vi "niRFUtil RFHS Math Complex Magnitude Squared.vi"(0 "data in":csg[](array[numeric]), 2 "RFHS?":bool=TRUE, 7 "result in":sgl[](array[numeric]), 11 "error in":errorcluster) -> (4 "result out":sgl[](array[numeric]), 15 "error out":errorcluster)   [LabVIEW 2015, in "niRFUtil.lvlib"]
uses:
  niRFUtil.lvlib
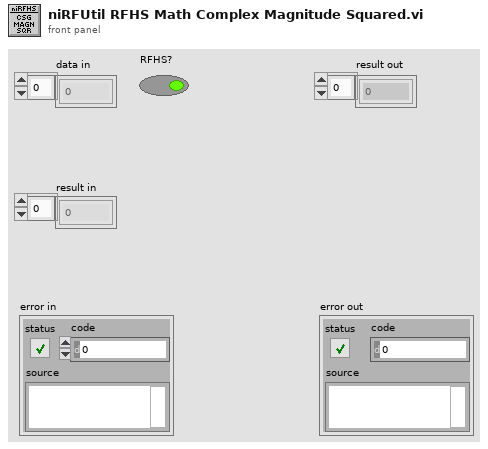
[diagram p1: front panel]
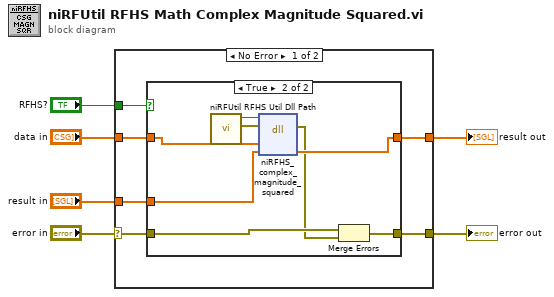
[diagram p0: block diagram]
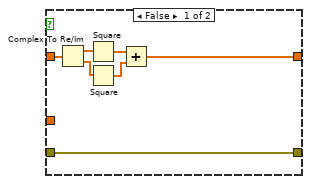
[diagram p2: hidden frame]
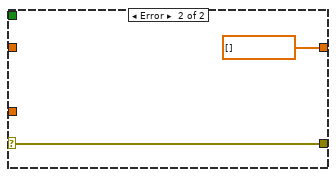
[diagram p3: hidden frame]
diagram:
  n1 = case shown="No Error" "error in" {
    selector: "error in" -> [w9 w29]
    tunnel: "RFHS?" -> [w12 _]
    tunnel: "data in" -> [w11 _]
    tunnel: [w10 sgl[] [] ("result")] -> w4
    tunnel: [w8 w29] -> w2
    tunnel: "result in" -> [w7 _]
    frame No Error {
      n2 = case shown="True" w12 {
        tunnel: w11 -> [w14 w27]
        tunnel: [w13 w26] -> w10
        tunnel: w9 -> [w19 w23]
        tunnel: [w19 w21] -> w8
        tunnel: w7 -> [_ w20]
        frame False {
          n3 = Complex To Re/Im(x + iy=w14) -> (x=w16:sgl[], y=w15:sgl[])
          n4 = Square(x=w16) -> (x^2=w18:sgl[])
          n5 = Square(x=w15) -> (x^2=w17:sgl[])
          n6 = Add(x=w18, y=w17) -> (x+y=w13:sgl[])
        }
        frame True {
          n7 = call "niRFUtil RFHS Util Dll Path.vi"() -> ("error out"=w25:errorcluster, "Path"=w24:path)  [unwired: 7 in, 3 out]
          n8 = dll-call lib="R:/niRFHS.dll" fn="niRFHS_complex_magnitude_squared"(path in=w24, error in=w25, "data"=w27, "result"=w20) -> (error out=w22:errorcluster, "result"=w26:sgl[])  [unwired: 3 in, 1 out]
          n9 = Merge Errors(w23, w22) -> (w21:errorcluster)
        }
      }
    }
    frame Error {
    }
  }
  "result out" <- w4
  "error out" <- w2
